vi "Check Connected Status.vi"(8 "Error In":errorcluster, 10 "Links":T1, 11 "WorkspaceManager in":T3) -> (0 "Error Out":errorcluster, 2 "Connected?":bool, 3 "WorkspaceManager out":T3)   [LabVIEW 2011]
uses:
  <vilib>/NI Veristand/Execution/Workspace/WorkspaceAPI.ctl
  NationalInstruments.VeriStand.ClientAPI
  Controls/Control Links.ctl
  Controls/ECUMC Item.ctl
  <vilib>/NI Veristand/Execution/Workspace/SystemState.ctl
  <vilib>/NI Veristand/Execution/Workspace/NI VeriStand - Get Multiple Channel Values.vi
  <vilib>/NI Veristand/Execution/Workspace/NI_VS Workspace ExecutionAPI.lvlib
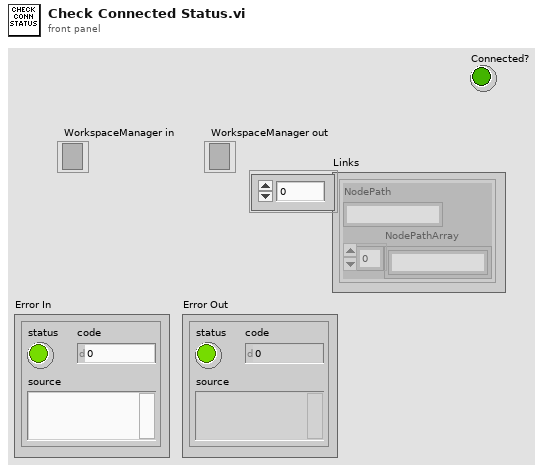
[diagram p1: front panel]
types:
  T1 = typedef "Control Links.ctl" = T2[]
  T2 = typedef "ECUMC Item.ctl" = cluster{"NodePath":string, "NodePathArray":string[]}
  T3 = typedef "NI_VS Workspace ExecutionAPI.lvlib/WorkspaceAPI.ctl" = refnum<k24>
  T4 = typedef "NI_VS Workspace ExecutionAPI.lvlib/SystemState.ctl" = u8
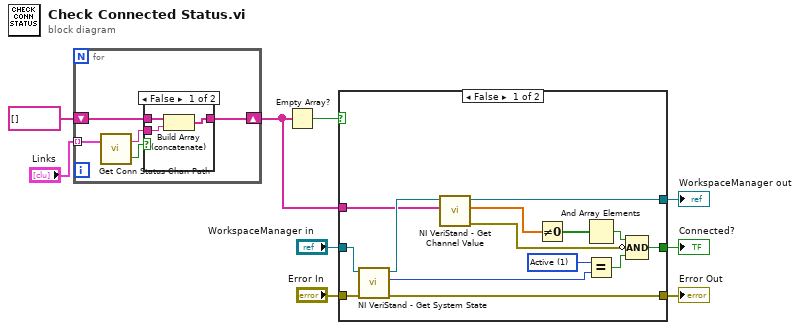
[diagram p0: block diagram]
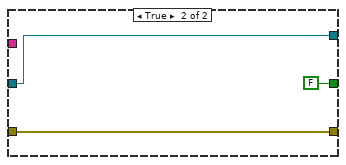
[diagram p2: hidden frame]
diagram:
  n1 = for {
    tunnel: "Links" -> [w14] mode=indexing
    shift-right: [w11] -> w1
    shift-left: string[] [] -> [w10]
    n2 = call "Get Conn Status Chan Path.vi"("Link"=w14) -> ("Empty Link?"=w13:bool, "Conn Status Chan"=w12:string)  [unwired: 1 in]
    n3 = case shown="False" w13 {
      tunnel: w12 -> [w17 _]
      tunnel: [w16 w18] -> w11
      tunnel: w10 -> [w15 w18]
      frame False {
        n4 = Build Array (concatenate)(w15, w17) -> (w16:string[])
      }
      frame True {
      }
    }
  }
  n5 = Empty Array?(array=w1) -> (empty?=w3:bool)
  n6 = case shown="False" w3 {
    tunnel: "Error In" -> [w30 w33]
    tunnel: "WorkspaceManager in" -> [w29 w34]
    tunnel: [w27 w34] -> w5
    tunnel: [w25 w33] -> w4
    tunnel: [w21 FALSE] -> w2
    tunnel: w1 -> [w26 _]
    frame False {
      w31 = T4 1 items=["Idle", "Active"] ("y")
      n7 = call <vilib>:"NI VeriStand - Get System State.vi"("error in (no error)"=w30, "WorkspaceManager in"=w29) -> ("error out"=w25:errorcluster, "System State"=w32:T4, "WorkspaceManager  out"=w28:T3)  [unwired: 5 in, 2 out]
      n8 = call-poly <vilib>:"NI VeriStand - Get Channel Value.vi"("Channels"=w26, "WorkspaceManager in"=w28) -> ("error out"=w20:errorcluster, "Values"=w24:dbl[], "WorkspaceManager out"=w27:T3)  [unwired: 7 in]
      n9 = Not Equal To 0?(x=w24) -> (x != 0?=w23:bool[])
      n10 = And Array Elements(Boolean array=w23) -> (logical AND=w22:bool)
      n11 = Equal?(x=w31, y=w32) -> (x = y?=w19:bool)
      n12 = Compound Arithmetic op=AND(w22, invert w20, w19) -> (w21:bool)
    }
    frame True {
    }
  }
  "Error Out" <- w4
  "WorkspaceManager out" <- w5
  "Connected?" <- w2
